vi "res_BATCH_offset.vi"(7 "Serialized by PLC? (F)":bool, 10 "ST_results_info":T1, 11 "BATCH_position":i32) -> (3 "results_byte_array_offset":i32)   [LabVIEW 2020]
uses:
  ST_results_info.ctl
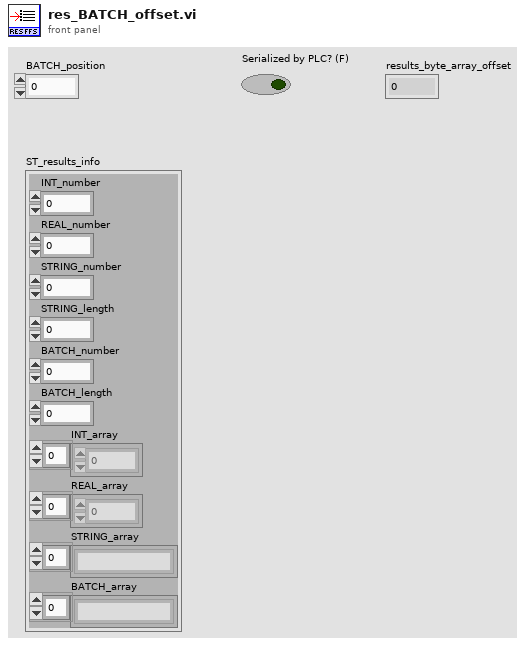
[diagram p1: front panel]
types:
  T1 = typedef "ST_results_info.ctl" = cluster{"INT_number":i32, "REAL_number":i32, "STRING_number":i32, "STRING_length":i32, "BATCH_number":i32, "BATCH_length":i32, "INT_array":i16[], "REAL_array":sgl[], "STRING_array":string[], "BATCH_array":string[]}
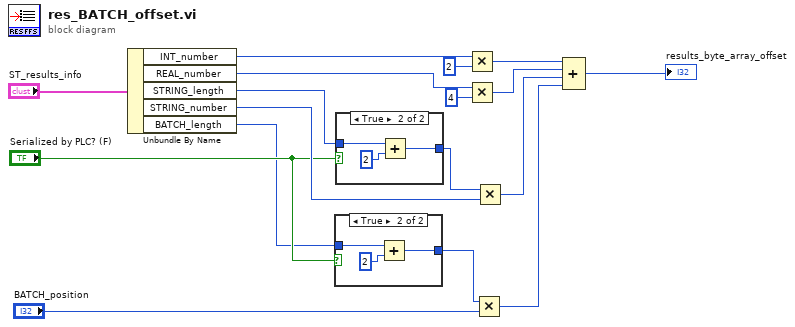
[diagram p0: block diagram]
diagram:
  n1 = Unbundle By Name("ST_results_info") -> ("INT_number"=w16:i32, "REAL_number"=w14:i32, "STRING_length"=w9:i32, "STRING_number"=w7:i32, "BATCH_length"=w5:i32)
  n2 = case shown="True" "Serialized by PLC? (F)" {
    tunnel: w5 -> [w18 w21]
    tunnel: [w18 w19] -> w4
    frame False {
    }
    frame True {
      n3 = Add(x=w21, y=2) -> (x+y=w19:i32)
    }
  }
  n4 = case shown="True" "Serialized by PLC? (F)" {
    tunnel: w9 -> [w22 w25]
    tunnel: [w22 w23] -> w8
    frame False {
    }
    frame True {
      n5 = Add(x=w25, y=2) -> (x+y=w23:i32)
    }
  }
  n6 = Multiply(x=w16, y=2) -> (x*y=w12:i32)
  n7 = Multiply(x=w14, y=4) -> (x*y=w11:i32)
  n8 = Multiply(x=w4, y="BATCH_position") -> (x*y=w2:i32)
  n9 = Multiply(x=w8, y=w7) -> (x*y=w10:i32)
  n10 = Compound Arithmetic op=ADD(w12, w11, w10, w2) -> (→"results_byte_array_offset":i32)
